vi "Process Array Elements (data types).vi"(0 "Queue In":refnum<queue>, 1 "Format String (%#0.15f)":string="%#0.15f", 5 "Array Variant":variant, 7 "Data type":variant, 9 "Name In":string, 11 "Error In":errorcluster) -> (4 "Queue Out":refnum<queue>, 10 "Data Out":string, 15 "Error Out":errorcluster)   [LabVIEW 2020]
doc: "This VI was created for use with the Read/Write Cluster VIs. It converts array elements of the cluster to strings to be written to file.\n\nFreeware from Moore Good Ideas, www.mooregoodideas.com. Do not remove this line."
uses:
  <vilib>/Utility/VariantDataType/VariantType.lvlib
  <vilib>/Utility/Data Type/NI_Data Type.lvlib
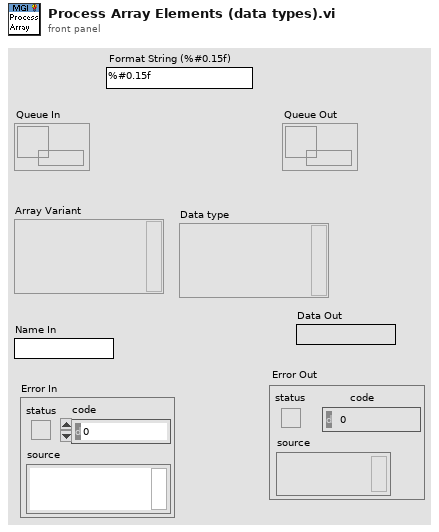
[diagram p1: front panel]
types:
  T1 = typedef "NI_Data Type.lvlib/Data Type.ctl" = enum8{"Invalid Type", "Void", "I8", "I16", "I32", "I64", "U8", "U16", "U32", "U64", "Single Float", "Double Float", "Extended Float", "Single Complex", "Double Complex", "Extended Complex", "Enum U8", "Enum U16", "Enum U32", "Enum U64", "Single Float With Unit", "Double Float With Unit", "Extended Float With Unit", "Single Complex with Unit", "Double Complex with Unit", "Extended Complex with Unit", "Boolean", "String", "Path", "Picture", "Tag", "Array", "Cluster", "Variant", "LV Variant", "Waveform", "Timestamp", "Digital Waveform", "Digital Data", "ExpressData", "Refnum", "External Data", "VI", "Poly VI", "LabVIEW Class Instance", "Fixed Point", "Set Collection", "Map Collection"}
  T2 = cluster{"Variant":variant, "array element data type":variant, "Name Out":string}
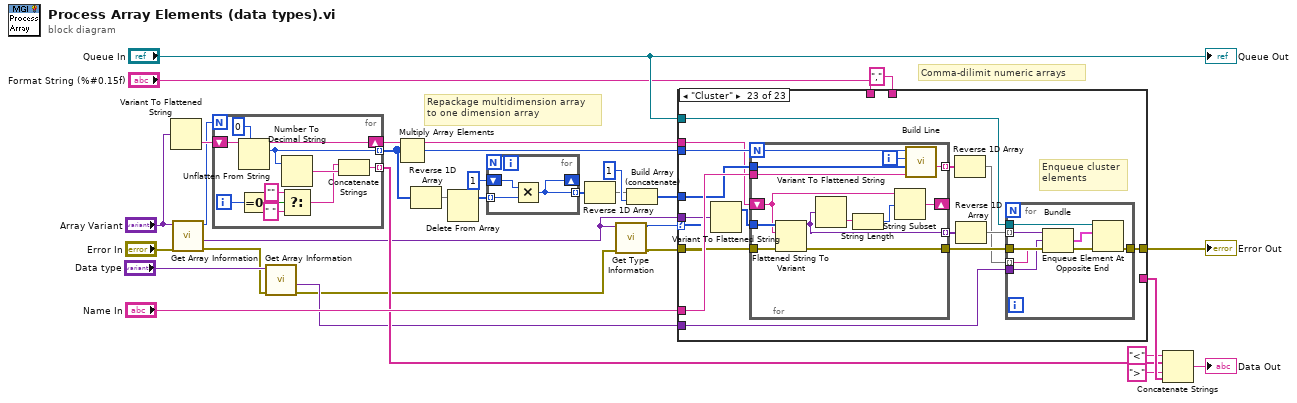
[diagram p0: block diagram]
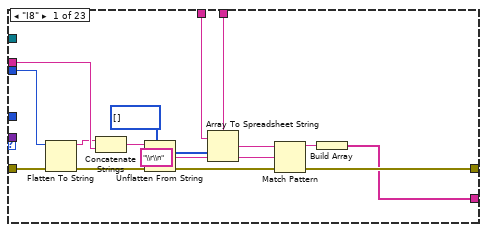
[diagram p2: hidden frame]
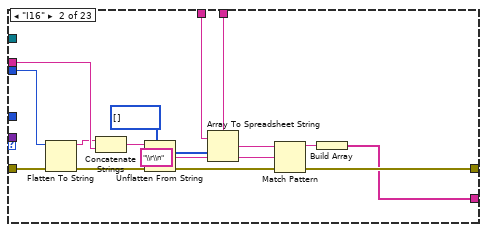
[diagram p3: hidden frame]
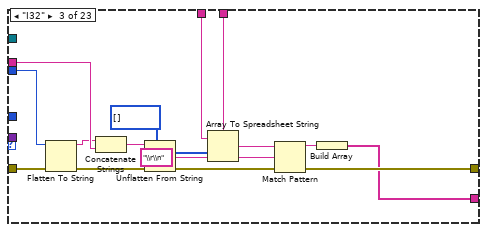
[diagram p4: hidden frame]
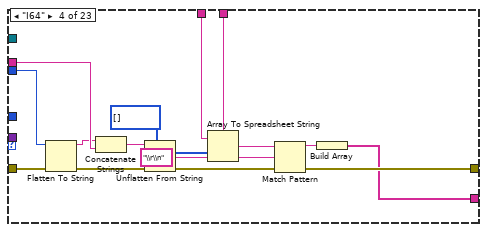
[diagram p5: hidden frame]
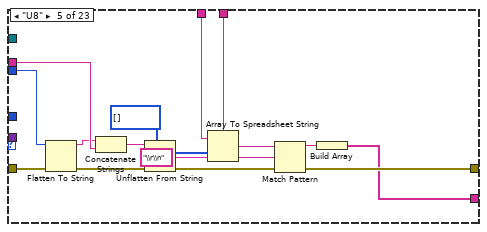
[diagram p6: hidden frame]
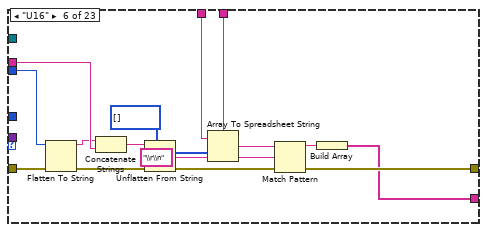
[diagram p7: hidden frame]
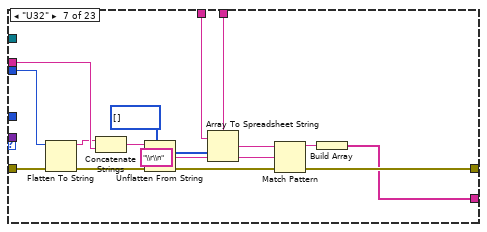
[diagram p8: hidden frame]
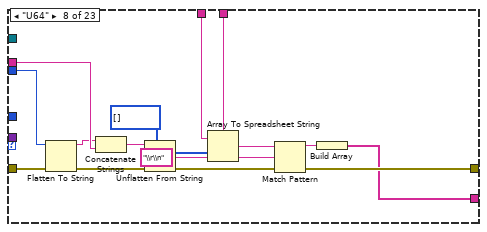
[diagram p9: hidden frame]
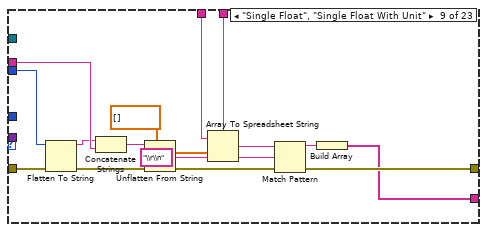
[diagram p10: hidden frame]
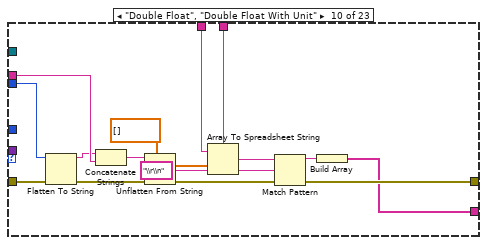
[diagram p11: hidden frame]
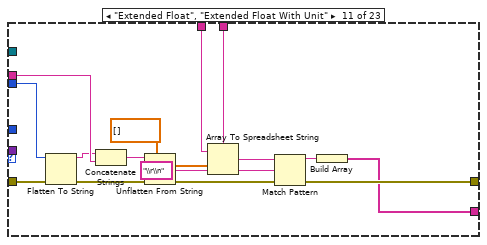
[diagram p12: hidden frame]
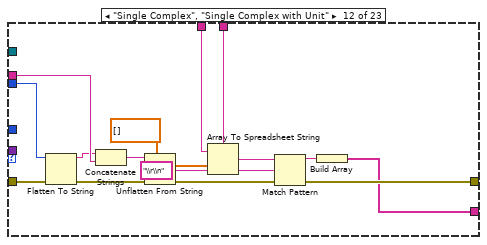
[diagram p13: hidden frame]
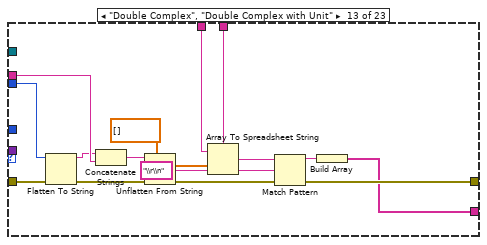
[diagram p14: hidden frame]
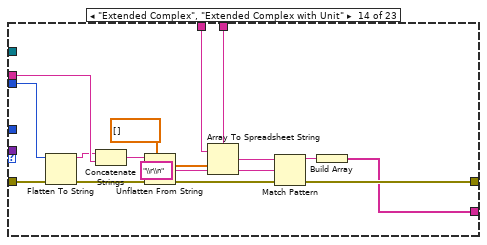
[diagram p15: hidden frame]
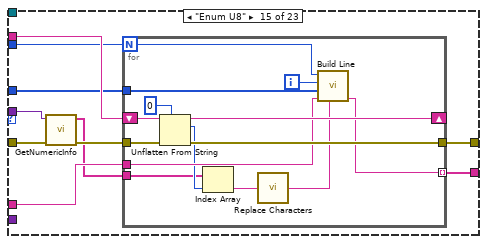
[diagram p16: hidden frame]
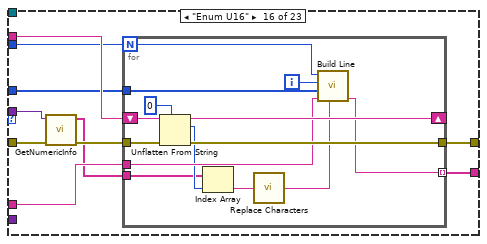
[diagram p17: hidden frame]
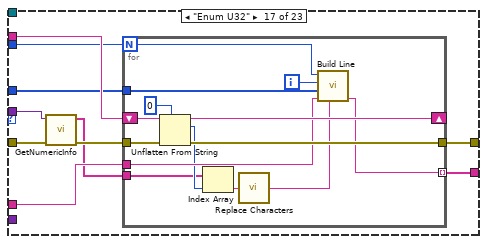
[diagram p18: hidden frame]
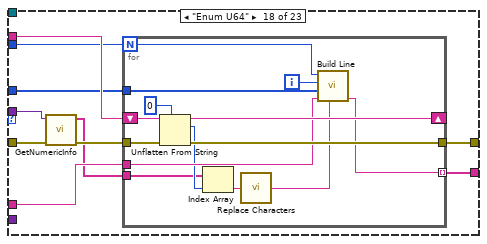
[diagram p19: hidden frame]
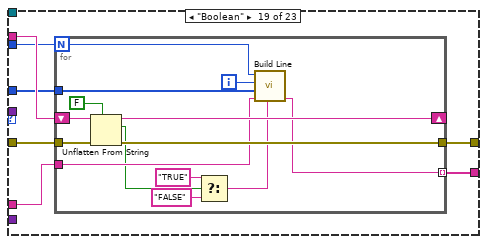
[diagram p20: hidden frame]
diagram:
  # "Comma-dilimit numeric arrays"
  # "Repackage multidimension array\nto one dimension array"
  n1 = Variant To Flattened String(Variant="Array Variant") -> (data string=w31:string)  [unwired: 1 out]
  n2 = call <vilib>:"Get Array Information.vi"("error in (no error)"="Error In", "variant"="Array Variant") -> ("error out"=w6:errorcluster, "array element data type"=w5:variant, "number of dimensions"=w9:i32)  [unwired: 6 in, 1 out]
  n3 = for {
    N: w9 -> [_]
    shift-right: [w40] -> w30
    shift-left: w31 -> [w41]
    tunnel: [w37] -> w19 mode=indexing
    tunnel: [w38] -> w15 mode=indexing
    i -> [w36]
    n4 = Unflatten From String(type=u32 0, binary string=w41) -> (rest of the binary string=w40:string, value=w37:u32)  [unwired: 3 in, 1 out]
    n5 = Equal To 0?(x=w36) -> (x = 0?=w35:bool)
    n6 = Number To Decimal String(number=w37) -> (decimal integer string=w39:string)  [unwired: 1 in]
    n7 = Select(t="", s=w35, f=" ") -> (s? t:f=w33:string)
    n8 = Concatenate Strings(w33, w39) -> (w38:string)
  }
  n9 = call <vilib>:"Get Array Information.vi"("error in (no error)"=w6, "variant"="Data type") -> ("error out"=w1:errorcluster, "array element data type"=w2:variant)  [unwired: 6 in, 2 out]
  n10 = Multiply Array Elements(1:w19) -> (0:w29:u32)
  n11 = Reverse 1D Array(array=w19) -> (reversed array=w20:u32[])
  n12 = Delete From Array(array=w20) -> (array with subset deleted=w21:u32[])  [unwired: 2 in, 1 out]
  n13 = for {
    tunnel: w21 -> [w45] mode=indexing
    shift-right: [w43] -> _
    shift-left: i8 1 -> [w44]
    tunnel: [w43] -> w23 mode=indexing
    n14 = Multiply(x=w44, y=w45) -> (x*y=w43:u32)
  }
  n15 = Reverse 1D Array(array=w23) -> (reversed array=w24:u32[])
  n16 = call <vilib>:"Get Type Information.vi"("error in (no error)"=w1, "variant"=w5) -> ("error out"=w3:errorcluster, "type"=w4:T1)  [unwired: 5 in, 3 out]
  n17 = Build Array (concatenate)(w24, i8 1) -> (w18:u32[])
  n18 = case shown="\"Cluster\"" w4 {
    tunnel: [w60 w75 w90 w105 w120 w135 w150 w165 w180 w195 w210 w225 w240 w255 w265 w289 w313 w337 w358 w379 w398 w414 w426] -> w17
    tunnel: w3 -> [w49 w64 w79 w94 w109 w124 w139 w154 w169 w184 w199 w214 w229 w244 w258 w282 w306 w330 w357 w378 w397 w414 w420]
    tunnel: w30 -> [w59 w74 w89 w104 w119 w134 w149 w164 w179 w194 w209 w224 w239 w254 w264 w288 w312 w336 w356 w377 w396 w413 w422]
    tunnel: w29 -> [w58 w73 w88 w103 w118 w133 w148 w163 w178 w193 w208 w223 w238 w253 w263 w287 w311 w335 w355 w376 w395 _ w433]
    tunnel: "Name In" -> [_ _ _ _ _ _ _ _ _ _ _ _ _ _ w262 w286 w310 w334 w354 w375 w394 _ w432]
    tunnel: [w57 w72 w87 w102 w117 w132 w147 w162 w177 w192 w207 w222 w237 w252 w260 w284 w308 w332 w352 w373 w392 w412 _] -> w27
    tunnel: w18 -> [_ _ _ _ _ _ _ _ _ _ _ _ _ _ w261 w285 w309 w333 w353 w374 w393 _ w431]
    tunnel: "Queue In" -> [_ _ _ _ _ _ _ _ _ _ _ _ _ _ _ _ _ _ _ _ _ _ w427]
    tunnel: w5 -> [_ _ _ _ _ _ _ _ _ _ _ _ _ _ w259 w283 w307 w331 _ _ _ _ w421]
    tunnel: "Format String (%#0.15f)" -> [w47 w62 w77 w92 w107 w122 w137 w152 w167 w182 w197 w212 w227 w242 _ _ _ _ _ _ _ _ _]
    tunnel: "," ("delimiter (Tab)") -> [w46 w61 w76 w91 w106 w121 w136 w151 w166 w181 w196 w211 w226 w241 _ _ _ _ _ _ _ _ _]
    tunnel: w2 -> [_ _ _ _ _ _ _ _ _ _ _ _ _ _ _ _ _ _ _ _ _ _ w419]
    frame "I8" {
      n19 = Flatten To String(anything=w58, error in (no error)=w49) -> (data string=w54:string, error out=w48:errorcluster)  [unwired: 2 in, 1 out]
      n20 = Concatenate Strings(w54, w59) -> (w55:string)
      n21 = Unflatten From String(type=i8[] [], binary string=w55, error in (no error)=w48) -> (value=w51:i8[], error out=w60:errorcluster)  [unwired: 2 in, 1 out]
      n22 = Array To Spreadsheet String(delimiter (Tab)=w46, array=w51, 3:w47) -> (spreadsheet string=w53:string)
      n23 = Match Pattern(string=w53, regular expression="\\r\\n") -> (before substring=w50:string)  [unwired: 1 in, 3 out]
      n24 = Build Array(w50) -> (w57:string[])
    }
    frame "I16" {
      n25 = Flatten To String(anything=w73, error in (no error)=w64) -> (data string=w69:string, error out=w63:errorcluster)  [unwired: 2 in, 1 out]
      n26 = Concatenate Strings(w69, w74) -> (w70:string)
      n27 = Unflatten From String(type=i16[] [], binary string=w70, error in (no error)=w63) -> (value=w66:i16[], error out=w75:errorcluster)  [unwired: 2 in, 1 out]
      n28 = Array To Spreadsheet String(delimiter (Tab)=w61, array=w66, 3:w62) -> (spreadsheet string=w68:string)
      n29 = Match Pattern(string=w68, regular expression="\\r\\n") -> (before substring=w65:string)  [unwired: 1 in, 3 out]
      n30 = Build Array(w65) -> (w72:string[])
    }
    frame "I32" {
      n31 = Flatten To String(anything=w88, error in (no error)=w79) -> (data string=w84:string, error out=w78:errorcluster)  [unwired: 2 in, 1 out]
      n32 = Concatenate Strings(w84, w89) -> (w85:string)
      n33 = Unflatten From String(type=i32[] [], binary string=w85, error in (no error)=w78) -> (value=w81:i32[], error out=w90:errorcluster)  [unwired: 2 in, 1 out]
      n34 = Array To Spreadsheet String(delimiter (Tab)=w76, array=w81, 3:w77) -> (spreadsheet string=w83:string)
      n35 = Match Pattern(string=w83, regular expression="\\r\\n") -> (before substring=w80:string)  [unwired: 1 in, 3 out]
      n36 = Build Array(w80) -> (w87:string[])
    }
    frame "I64" {
      n37 = Flatten To String(anything=w103, error in (no error)=w94) -> (data string=w99:string, error out=w93:errorcluster)  [unwired: 2 in, 1 out]
      n38 = Concatenate Strings(w99, w104) -> (w100:string)
      n39 = Unflatten From String(type=i64[] [], binary string=w100, error in (no error)=w93) -> (value=w96:i64[], error out=w105:errorcluster)  [unwired: 2 in, 1 out]
      n40 = Array To Spreadsheet String(delimiter (Tab)=w91, array=w96, 3:w92) -> (spreadsheet string=w98:string)
      n41 = Match Pattern(string=w98, regular expression="\\r\\n") -> (before substring=w95:string)  [unwired: 1 in, 3 out]
      n42 = Build Array(w95) -> (w102:string[])
    }
    frame "U8" {
      n43 = Flatten To String(anything=w118, error in (no error)=w109) -> (data string=w114:string, error out=w108:errorcluster)  [unwired: 2 in, 1 out]
      n44 = Concatenate Strings(w114, w119) -> (w115:string)
      n45 = Unflatten From String(type=u8[] [], binary string=w115, error in (no error)=w108) -> (value=w111:u8[], error out=w120:errorcluster)  [unwired: 2 in, 1 out]
      n46 = Array To Spreadsheet String(delimiter (Tab)=w106, array=w111, 3:w107) -> (spreadsheet string=w113:string)
      n47 = Match Pattern(string=w113, regular expression="\\r\\n") -> (before substring=w110:string)  [unwired: 1 in, 3 out]
      n48 = Build Array(w110) -> (w117:string[])
    }
    frame "U16" {
      n49 = Flatten To String(anything=w133, error in (no error)=w124) -> (data string=w129:string, error out=w123:errorcluster)  [unwired: 2 in, 1 out]
      n50 = Concatenate Strings(w129, w134) -> (w130:string)
      n51 = Unflatten From String(type=u16[] [], binary string=w130, error in (no error)=w123) -> (value=w126:u16[], error out=w135:errorcluster)  [unwired: 2 in, 1 out]
      n52 = Array To Spreadsheet String(delimiter (Tab)=w121, array=w126, 3:w122) -> (spreadsheet string=w128:string)
      n53 = Match Pattern(string=w128, regular expression="\\r\\n") -> (before substring=w125:string)  [unwired: 1 in, 3 out]
      n54 = Build Array(w125) -> (w132:string[])
    }
    frame "U32" {
      n55 = Flatten To String(anything=w148, error in (no error)=w139) -> (data string=w144:string, error out=w138:errorcluster)  [unwired: 2 in, 1 out]
      n56 = Concatenate Strings(w144, w149) -> (w145:string)
      n57 = Unflatten From String(type=u32[] [], binary string=w145, error in (no error)=w138) -> (value=w141:u32[], error out=w150:errorcluster)  [unwired: 2 in, 1 out]
      n58 = Array To Spreadsheet String(delimiter (Tab)=w136, array=w141, 3:w137) -> (spreadsheet string=w143:string)
      n59 = Match Pattern(string=w143, regular expression="\\r\\n") -> (before substring=w140:string)  [unwired: 1 in, 3 out]
      n60 = Build Array(w140) -> (w147:string[])
    }
    frame "U64" {
      n61 = Flatten To String(anything=w163, error in (no error)=w154) -> (data string=w159:string, error out=w153:errorcluster)  [unwired: 2 in, 1 out]
      n62 = Concatenate Strings(w159, w164) -> (w160:string)
      n63 = Unflatten From String(type=u64[] [], binary string=w160, error in (no error)=w153) -> (value=w156:u64[], error out=w165:errorcluster)  [unwired: 2 in, 1 out]
      n64 = Array To Spreadsheet String(delimiter (Tab)=w151, array=w156, 3:w152) -> (spreadsheet string=w158:string)
      n65 = Match Pattern(string=w158, regular expression="\\r\\n") -> (before substring=w155:string)  [unwired: 1 in, 3 out]
      n66 = Build Array(w155) -> (w162:string[])
    }
    frame "Single Float", "Single Float With Unit" {
      n67 = Flatten To String(anything=w178, error in (no error)=w169) -> (data string=w174:string, error out=w168:errorcluster)  [unwired: 2 in, 1 out]
      n68 = Concatenate Strings(w174, w179) -> (w175:string)
      n69 = Unflatten From String(type=sgl[] [], binary string=w175, error in (no error)=w168) -> (value=w171:sgl[], error out=w180:errorcluster)  [unwired: 2 in, 1 out]
      n70 = Array To Spreadsheet String(delimiter (Tab)=w166, array=w171, 3:w167) -> (spreadsheet string=w173:string)
      n71 = Match Pattern(string=w173, regular expression="\\r\\n") -> (before substring=w170:string)  [unwired: 1 in, 3 out]
      n72 = Build Array(w170) -> (w177:string[])
    }
    frame "Double Float", "Double Float With Unit" {
      n73 = Flatten To String(anything=w193, error in (no error)=w184) -> (data string=w189:string, error out=w183:errorcluster)  [unwired: 2 in, 1 out]
      n74 = Concatenate Strings(w189, w194) -> (w190:string)
      n75 = Unflatten From String(type=dbl[] [], binary string=w190, error in (no error)=w183) -> (value=w186:dbl[], error out=w195:errorcluster)  [unwired: 2 in, 1 out]
      n76 = Array To Spreadsheet String(delimiter (Tab)=w181, array=w186, 3:w182) -> (spreadsheet string=w188:string)
      n77 = Match Pattern(string=w188, regular expression="\\r\\n") -> (before substring=w185:string)  [unwired: 1 in, 3 out]
      n78 = Build Array(w185) -> (w192:string[])
    }
    frame "Extended Float", "Extended Float With Unit" {
      n79 = Flatten To String(anything=w208, error in (no error)=w199) -> (data string=w204:string, error out=w198:errorcluster)  [unwired: 2 in, 1 out]
      n80 = Concatenate Strings(w204, w209) -> (w205:string)
      n81 = Unflatten From String(type=ext[] [], binary string=w205, error in (no error)=w198) -> (value=w201:ext[], error out=w210:errorcluster)  [unwired: 2 in, 1 out]
      n82 = Array To Spreadsheet String(delimiter (Tab)=w196, array=w201, 3:w197) -> (spreadsheet string=w203:string)
      n83 = Match Pattern(string=w203, regular expression="\\r\\n") -> (before substring=w200:string)  [unwired: 1 in, 3 out]
      n84 = Build Array(w200) -> (w207:string[])
    }
    frame "Single Complex", "Single Complex with Unit" {
      n85 = Flatten To String(anything=w223, error in (no error)=w214) -> (data string=w219:string, error out=w213:errorcluster)  [unwired: 2 in, 1 out]
      n86 = Concatenate Strings(w219, w224) -> (w220:string)
      n87 = Unflatten From String(type=csg[] [], binary string=w220, error in (no error)=w213) -> (value=w216:csg[], error out=w225:errorcluster)  [unwired: 2 in, 1 out]
      n88 = Array To Spreadsheet String(delimiter (Tab)=w211, array=w216, 3:w212) -> (spreadsheet string=w218:string)
      n89 = Match Pattern(string=w218, regular expression="\\r\\n") -> (before substring=w215:string)  [unwired: 1 in, 3 out]
      n90 = Build Array(w215) -> (w222:string[])
    }
    frame "Double Complex", "Double Complex with Unit" {
      n91 = Flatten To String(anything=w238, error in (no error)=w229) -> (data string=w234:string, error out=w228:errorcluster)  [unwired: 2 in, 1 out]
      n92 = Concatenate Strings(w234, w239) -> (w235:string)
      n93 = Unflatten From String(type=cdb[] [], binary string=w235, error in (no error)=w228) -> (value=w231:cdb[], error out=w240:errorcluster)  [unwired: 2 in, 1 out]
      n94 = Array To Spreadsheet String(delimiter (Tab)=w226, array=w231, 3:w227) -> (spreadsheet string=w233:string)
      n95 = Match Pattern(string=w233, regular expression="\\r\\n") -> (before substring=w230:string)  [unwired: 1 in, 3 out]
      n96 = Build Array(w230) -> (w237:string[])
    }
    frame "Extended Complex", "Extended Complex with Unit" {
      n97 = Flatten To String(anything=w253, error in (no error)=w244) -> (data string=w249:string, error out=w243:errorcluster)  [unwired: 2 in, 1 out]
      n98 = Concatenate Strings(w249, w254) -> (w250:string)
      n99 = Unflatten From String(type=cxt[] [], binary string=w250, error in (no error)=w243) -> (value=w246:cxt[], error out=w255:errorcluster)  [unwired: 2 in, 1 out]
      n100 = Array To Spreadsheet String(delimiter (Tab)=w241, array=w246, 3:w242) -> (spreadsheet string=w248:string)
      n101 = Match Pattern(string=w248, regular expression="\\r\\n") -> (before substring=w245:string)  [unwired: 1 in, 3 out]
      n102 = Build Array(w245) -> (w252:string[])
    }
    frame "Enum U8" {
      n103 = call <vilib>:"GetNumericInfo.vi"("error in (no error)"=w258, "Variant"=w259) -> ("error out"=w257:errorcluster, "EnumNames"=w256:string[])  [unwired: 6 in, 2 out]
      n104 = for {
        N: w263 -> [w275]
        tunnel: [w276] -> w265
        tunnel: w257 -> [w277]
        shift-right: [w278] -> _
        shift-left: w264 -> [w279]
        tunnel: w262 -> [w271]
        tunnel: [w272] -> w260 mode=indexing
        tunnel: w261 -> [w273]
        tunnel: w256 -> [w268]
        i -> [w274]
        n105 = Unflatten From String(type=u8 0, binary string=w279, error in (no error)=w277) -> (rest of the binary string=w278:string, value=w269:u8, error out=w276:errorcluster)  [unwired: 2 in]
        n106 = Index Array(array=w268, index=w269) -> (element=w267:string)
        n107 = call "Replace Characters.vi"("String In"=w267) -> ("String Out"=w266:string)  [unwired: 1 in]
        n108 = call "Build Line.vi"("Value String (\"\")"=w266, "Name In"=w271, "Array"=w273, "Iteration"=w274, "Iterations"=w275) -> ("Line"=w272:string)  [unwired: 5 in, 1 out]
      }
    }
    frame "Enum U16" {
      n109 = call <vilib>:"GetNumericInfo.vi"("error in (no error)"=w282, "Variant"=w283) -> ("error out"=w281:errorcluster, "EnumNames"=w280:string[])  [unwired: 6 in, 2 out]
      n110 = for {
        N: w287 -> [w299]
        tunnel: [w300] -> w289
        tunnel: w281 -> [w301]
        shift-right: [w302] -> _
        shift-left: w288 -> [w303]
        tunnel: w286 -> [w295]
        tunnel: [w296] -> w284 mode=indexing
        tunnel: w285 -> [w297]
        tunnel: w280 -> [w292]
        i -> [w298]
        n111 = Unflatten From String(type=u16 0, binary string=w303, error in (no error)=w301) -> (rest of the binary string=w302:string, value=w293:u16, error out=w300:errorcluster)  [unwired: 2 in]
        n112 = Index Array(array=w292, index=w293) -> (element=w291:string)
        n113 = call "Replace Characters.vi"("String In"=w291) -> ("String Out"=w290:string)  [unwired: 1 in]
        n114 = call "Build Line.vi"("Value String (\"\")"=w290, "Name In"=w295, "Array"=w297, "Iteration"=w298, "Iterations"=w299) -> ("Line"=w296:string)  [unwired: 5 in, 1 out]
      }
    }
    frame "Enum U32" {
      n115 = call <vilib>:"GetNumericInfo.vi"("error in (no error)"=w306, "Variant"=w307) -> ("error out"=w305:errorcluster, "EnumNames"=w304:string[])  [unwired: 6 in, 2 out]
      n116 = for {
        N: w311 -> [w323]
        tunnel: [w324] -> w313
        tunnel: w305 -> [w325]
        shift-right: [w326] -> _
        shift-left: w312 -> [w327]
        tunnel: w310 -> [w319]
        tunnel: [w320] -> w308 mode=indexing
        tunnel: w309 -> [w321]
        tunnel: w304 -> [w316]
        i -> [w322]
        n117 = Unflatten From String(type=u32 0, binary string=w327, error in (no error)=w325) -> (rest of the binary string=w326:string, value=w317:u32, error out=w324:errorcluster)  [unwired: 2 in]
        n118 = Index Array(array=w316, index=w317) -> (element=w315:string)
        n119 = call "Replace Characters.vi"("String In"=w315) -> ("String Out"=w314:string)  [unwired: 1 in]
        n120 = call "Build Line.vi"("Value String (\"\")"=w314, "Name In"=w319, "Array"=w321, "Iteration"=w322, "Iterations"=w323) -> ("Line"=w320:string)  [unwired: 5 in, 1 out]
      }
    }
    frame "Enum U64" {
      n121 = call <vilib>:"GetNumericInfo.vi"("error in (no error)"=w330, "Variant"=w331) -> ("error out"=w329:errorcluster, "EnumNames"=w328:string[])  [unwired: 6 in, 2 out]
      n122 = for {
        N: w335 -> [w347]
        tunnel: [w348] -> w337
        tunnel: w329 -> [w349]
        shift-right: [w350] -> _
        shift-left: w336 -> [w351]
        tunnel: w334 -> [w343]
        tunnel: [w344] -> w332 mode=indexing
        tunnel: w333 -> [w345]
        tunnel: w328 -> [w340]
        i -> [w346]
        n123 = Unflatten From String(type=u64 0, binary string=w351, error in (no error)=w349) -> (rest of the binary string=w350:string, value=w341:u64, error out=w348:errorcluster)  [unwired: 2 in]
        n124 = Index Array(array=w340, index=w341) -> (element=w339:string)
        n125 = call "Replace Characters.vi"("String In"=w339) -> ("String Out"=w338:string)  [unwired: 1 in]
        n126 = call "Build Line.vi"("Value String (\"\")"=w338, "Name In"=w343, "Array"=w345, "Iteration"=w346, "Iterations"=w347) -> ("Line"=w344:string)  [unwired: 5 in, 1 out]
      }
    }
    frame "Boolean" {
      n127 = for {
        N: w355 -> [w368]
        tunnel: [w369] -> w358
        tunnel: w357 -> [w370]
        shift-right: [w371] -> _
        shift-left: w356 -> [w372]
        tunnel: w354 -> [w364]
        tunnel: [w365] -> w352 mode=indexing
        tunnel: w353 -> [w366]
        i -> [w367]
        n128 = Unflatten From String(type=FALSE, binary string=w372, error in (no error)=w370) -> (rest of the binary string=w371:string, value=w360:bool, error out=w369:errorcluster)  [unwired: 2 in]
        n129 = Select(t="TRUE", s=w360, f="FALSE") -> (s? t:f=w359:string)
        n130 = call "Build Line.vi"("Value String (\"\")"=w359, "Name In"=w364, "Array"=w366, "Iteration"=w367, "Iterations"=w368) -> ("Line"=w365:string)  [unwired: 5 in, 1 out]
      }
    }
    frame "String" {
      n131 = for {
        N: w376 -> [w387]
        tunnel: [w388] -> w379
        tunnel: w378 -> [w389]
        shift-right: [w390] -> _
        shift-left: w377 -> [w391]
        tunnel: w375 -> [w383]
        tunnel: [w384] -> w373 mode=indexing
        tunnel: w374 -> [w385]
        i -> [w386]
        n132 = Unflatten From String(type="", binary string=w391, error in (no error)=w389) -> (rest of the binary string=w390:string, value=w381:string, error out=w388:errorcluster)  [unwired: 2 in]
        n133 = call "Replace Characters.vi"("String In"=w381) -> ("String Out"=w380:string)  [unwired: 1 in]
        n134 = call "Build Line.vi"("Value String (\"\")"=w380, "Name In"=w383, "Array"=w385, "Iteration"=w386, "Iterations"=w387) -> ("Line"=w384:string)  [unwired: 5 in, 1 out]
      }
    }
    frame "Path" {
      n135 = for {
        N: w395 -> [w407]
        tunnel: [w408] -> w398
        tunnel: w397 -> [w409]
        shift-right: [w410] -> _
        shift-left: w396 -> [w411]
        tunnel: w394 -> [w403]
        tunnel: [w404] -> w392 mode=indexing
        tunnel: w393 -> [w405]
        i -> [w406]
        n136 = Unflatten From String(type=path "", binary string=w411, error in (no error)=w409) -> (rest of the binary string=w410:string, value=w401:path, error out=w408:errorcluster)  [unwired: 2 in]
        n137 = Path To String(path=w401) -> (string=w400:string)
        n138 = call "Replace Characters.vi"("String In"=w400) -> ("String Out"=w399:string)  [unwired: 1 in]
        n139 = call "Build Line.vi"("Value String (\"\")"=w399, "Name In"=w403, "Array"=w405, "Iteration"=w406, "Iterations"=w407) -> ("Line"=w404:string)  [unwired: 5 in, 1 out]
      }
    }
    frame Default {
      n140 = String To Byte Array(string=w413) -> (unsigned byte array=w418:u8[])
      n141 = Number To Hexadecimal String(1:i16 2 ("width (-)"), 2:w418) -> (0:w417:string[])
      n142 = Build Array (concatenate)("0x", w417) -> (w412:string[])
    }
    frame "Cluster" {
      # "Enqueue cluster\nelements"
      n143 = Variant To Flattened String(Variant=w421) -> (1:w424:i16[])  [unwired: 1 out]
      n144 = for {
        N: w433 -> [w453]
        tunnel: [w447] -> w428
        tunnel: w420 -> [w449]
        tunnel: w432 -> [w445]
        tunnel: w431 -> [w451]
        tunnel: [w441] -> w429 mode=indexing
        tunnel: [w450] -> w425 mode=indexing
        tunnel: w424 -> [w448]
        shift-right: [w442] -> _
        shift-left: w422 -> [w443]
        i -> [w452]
        n145 = Flattened String To Variant(4:w449, 6:w443, 7:w448) -> (0:w447:errorcluster, 3:w441:variant)
        n146 = Variant To Flattened String(Variant=w441) -> (data string=w446:string)  [unwired: 1 out]
        n147 = String Length(string=w446) -> (length=w444:i32)
        n148 = String Subset(string=w443, offset (0)=w444) -> (substring=w442:string)  [unwired: 1 in]
        n149 = call "Build Line.vi"("Name In"=w445, "Array"=w451, "Iteration"=w452, "Iterations"=w453) -> ("Name Out"=w450:string)  [unwired: 6 in, 1 out]
      }
      n150 = Reverse 1D Array(array=w425) -> (reversed array=w423:string[])
      n151 = Reverse 1D Array(array=w429) -> (reversed array=w430:variant[])
      n152 = for {
        tunnel: [w440] -> w426
        tunnel: w430 -> [w439] mode=indexing
        tunnel: w428 -> [w438]
        tunnel: w427 -> [w437]
        tunnel: w423 -> [w436] mode=indexing
        tunnel: w419 -> [w435]
        n153 = Bundle("Variant"=w439, "array element data type"=w435, "Name Out"=w436) -> (w434:T2)  [unwired: 1 in]
        n154 = Enqueue Element At Opposite End(queue=w437, element=w434, error in (no error)=w438) -> (error out=w440:errorcluster)  [unwired: 1 in, 2 out]
      }
    }
  }
  "Error Out" <- w17
  n155 = Concatenate Strings("<", w15, ">", w27) -> (→"Data Out":string)
  "Queue Out" <- "Queue In"
